vi "Temperature Write Single.vi"(8 "error in":errorcluster, 9 "Channel Index":i32=1, 10 "Temperature AV":dbl, 11 "Chiller in":refnum<class "Chiller.lvclass">) -> (0 "error out":errorcluster, 3 "Chiller out":refnum<class "Chiller.lvclass">)   [LabVIEW 2023, in "Chiller.lvclass"]
uses:
  Chiller.lvclass
  Chiller.lvclass/Chiller.ctl
  Low Level Capabilities/Temperature/Temperature Actual Value/Temperature Actual Value.lvclass
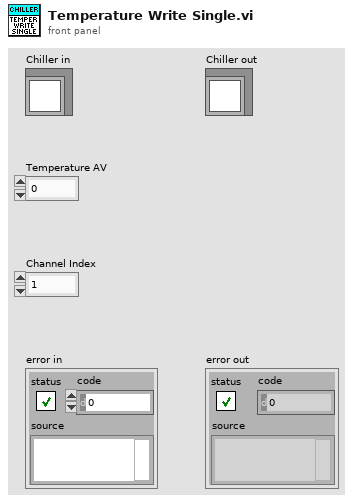
[diagram p1: front panel]
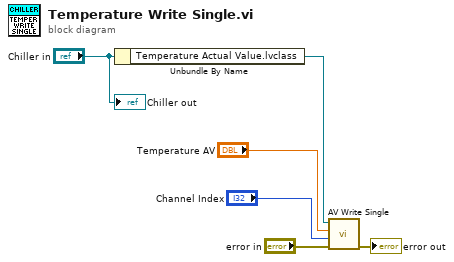
[diagram p0: block diagram]
diagram:
  n1 = Unbundle By Name("Chiller in") -> ("Temperature Actual Value.lvclass"=w6:refnum<class "Temperature Actual Value.lvclass">)
  n2 = call-dynamic "AV Write Single.vi"("error in"="error in", "Channel Index"="Channel Index", "Temperature AV"="Temperature AV", "Temperature Actual Value in"=w6) -> ("error out"=→"error out":errorcluster)  [unwired: 6 in, 1 out]
  "Chiller out" <- "Chiller in"
